vi "VALEW_Sensors_Hall.vi"(0 "GEA2 Reference In":refnum<k24>, 5 "GEA Inputs":T1={"Source"=228, "Destination"=35} {"Destination" format="%.0x"; "Source" format="%.0x"}, 7 "DAQmx Physical Channel":tag="9401_1/ctr2", 9 "Counter Terminal":tag="/9401_1/PFI4", 11 "Error In":errorcluster, 12 "Basket Test RPMs":dbl[](array[numeric])=[125.0, 500.0, 700.0], 13 "Max Error (RPM)":dbl=3.0, 14 "Standalone?":bool=TRUE) -> (4 "GEA2 Reference Out":refnum<k24>, 6 "Pass/Fail?":bool, 8 "Report Text":string, 15 "Error Out":errorcluster)   [LabVIEW 2016, in "2015 VA Washer.lvlib"]
doc: "This VI outputs the Test RPMs by generating a frequency that is 0.3 * Test RPM Value and verifies the Basket speed ERD is within the Max Error defined."
uses:
  Projects/2015 VA Washer.lvlib
  C:/Automation/DLLs/PC Dot Net/GeaCommunication.dll
  Common/LabVIEW GEA2 Toolkit/LabVIEW_GEA2_Toolkit.lvlibp/type defs/Source_Destination.ctl
  Common/LabVIEW GEA2 Toolkit/LabVIEW_GEA2_Toolkit.lvlibp/type defs/ERD Read Data In.ctl
  Common/LabVIEW GEA2 Toolkit/LabVIEW_GEA2_Toolkit.lvlibp/type defs/Data Type.ctl
  <vilib>/DAQmx/create/channels.llb/DAQmx Create Channel (CO-Pulse Generation-Frequency).vi
  <vilib>/DAQmx/configure/timing.llb/DAQmx Timing (Implicit).vi
  Common/LabVIEW GEA2 Toolkit/LabVIEW_GEA2_Toolkit.lvlibp
  <resource>/objmgr/daqmx.rc
panel:
  out "Lim_U_Basket Speed RPM":dbl[](array[numeric])
  out "Lim_L_Basket Speed RPM":dbl[](array[numeric])
  out "Basket Speed RPM":dbl[](array[numeric])
  out "Lim_L_Shaft Speed RPM":dbl[](array[numeric])
  out "Lim_U_Shaft Speed RPM":dbl[](array[numeric])
  out "Shaft Speed RPM":dbl[](array[numeric])
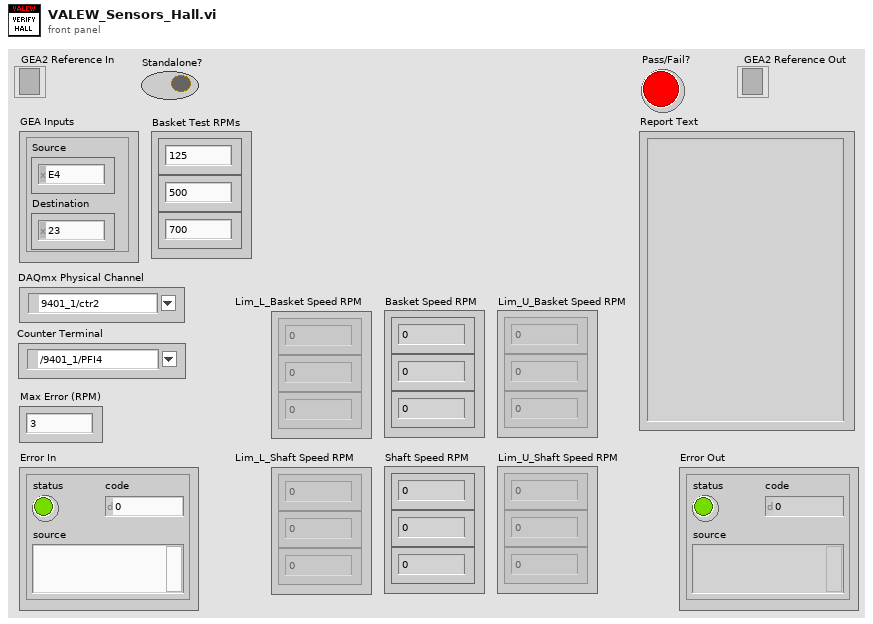
[diagram p1: front panel]
types:
  T1 = typedef "LabVIEW_GEA2_Toolkit.lvlibp/Source_Destination.ctl" = cluster{"Source":u8, "Destination":u8}
  T2 = typedef "LabVIEW_GEA2_Toolkit.lvlibp/ERD Read Data In.ctl" = cluster{"ERD Number":u16, "Data Type":T3}
  T3 = typedef "LabVIEW_GEA2_Toolkit.lvlibp/Data Type.ctl" = enum16{"string", "boolean", "uint8_t", "uint16_t", "uint32_t", "uint64_t", "int8_t", "int16_t", "int32_t", "int64_t"}
  T4 = typedef "LabVIEW_GEA2_Toolkit.lvlibp/ERD Read Data Out.ctl" = cluster{"ERD Number":u16, "Data":string}
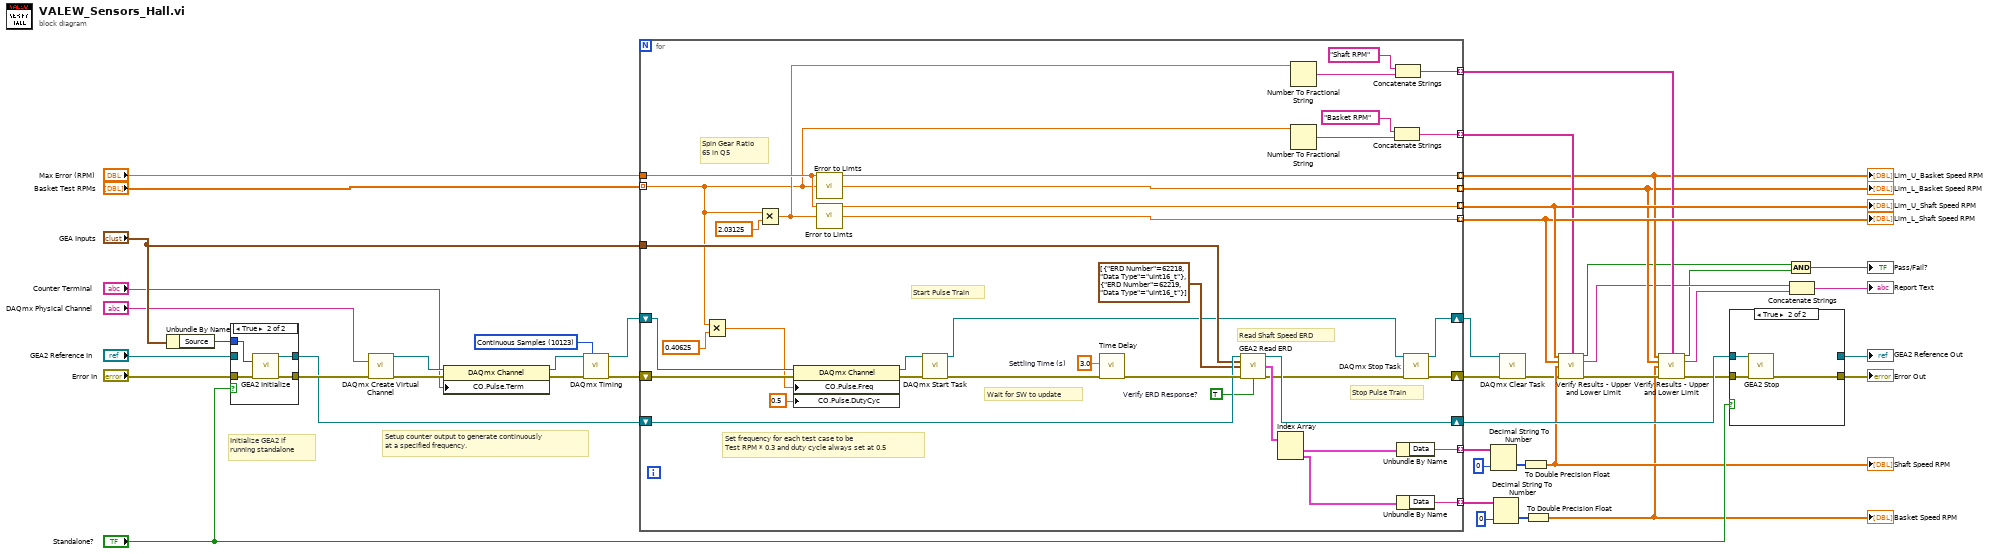
[diagram p0: block diagram]
diagram:
  w26 = 10123 items=["Finite Samples"=10178, "Continuous Samples"=10123, "Hardware Timed Single Point"=12522] ("sample mode")
  # "Setup counter output to generate continuously\nat a specified frequency."
  # "Initialize GEA2 if\nrunning standalone"
  n1 = Unbundle By Name("GEA Inputs") -> ("Source"=w38:u8)
  n2 = case shown="True" "Standalone?" {
    tunnel: "Error In" -> [w48 w52]
    tunnel: [w48 w51] -> w44
    tunnel: "GEA2 Reference In" -> [w47 _]
    tunnel: [w47 w50] -> w40
    tunnel: w38 -> [_ w49]
    frame False {
    }
    frame True {
      n3 = call "GEA2 Initialize.vi"("Source Address"=w49, "error in"=w52) -> ("GEA2 Reference Out"=w50:refnum<k24>, "error out"=w51:errorcluster)  [unwired: 11 in, 1 out]
    }
  }
  n4 = call-poly <vilib>:"DAQmx Create Virtual Channel.vi"("counter"="DAQmx Physical Channel", "error in"=w44) -> ("task out"=w31:refnum<k21>, "error out"=w32:errorcluster)  [unwired: 12 in]
  n5 = property class="DAQmx Channel"(reference=w31, error in=w32, "CO.Pulse.Term"="Counter Terminal") -> (reference out=w27:refnum<k21>, error out=w24:errorcluster)
  n6 = call-poly <vilib>:"DAQmx Timing.vi"("task/channels in"=w27, "sample mode"=w26, "error in"=w24) -> ("task out"=w25:refnum<k21>, "error out"=w23:errorcluster)  [unwired: 11 in]
  n7 = for {
    shift-right: [w79] -> w39
    shift-left: w40 -> [w88]
    shift-right: [w72] -> w43
    shift-left: w25 -> [w82]
    shift-right: [w73] -> w2
    shift-left: w23 -> [w81]
    tunnel: "GEA Inputs" -> [w87]
    tunnel: [w84] -> w36 mode=indexing
    tunnel: "Basket Test RPMs" -> [w53] mode=indexing
    tunnel: "Max Error (RPM)" -> [w60]
    tunnel: [w71] -> w20 mode=indexing
    tunnel: [w70] -> w21 mode=indexing
    tunnel: [w67] -> w18 mode=indexing
    tunnel: [w62] -> w12 mode=indexing
    tunnel: [w61] -> w11 mode=indexing
    tunnel: [w58] -> w15 mode=indexing
    tunnel: [w55] -> w13 mode=indexing
    w83 = TRUE  # Verify ERD Response?
    w90 = 3.0  # Settling Time (s)
    # "Spin Gear Ratio\n65 in Q5"
    # "Stop Pulse Train"
    # "Read Shaft Speed ERD"
    # "Wait for SW to update"
    # "Start Pulse Train"
    # "Set frequency for each test case to be\nTest RPM * 0.3 and duty cycle always set at 0.5"
    n8 = Multiply(x=w53, y=0.40625) -> (x*y=w63:dbl)
    n9 = Multiply(x=w53, y=2.03125) -> (x*y=w54:dbl)
    n10 = property class="DAQmx Channel"(reference=w82, error in=w81, "CO.Pulse.Freq"=w63, "CO.Pulse.DutyCyc"=0.5) -> (reference out=w75:refnum<k21>, error out=w76:errorcluster)
    n11 = call "Error to Limts.vi"("Error"=w60, "Value"=w53) -> ("Upper Limit"=w62:dbl, "Lower Limit"=w61:dbl)  [unwired: 12 in]
    n12 = call "Error to Limts.vi"("Error"=w60, "Value"=w54) -> ("Upper Limit"=w70:dbl, "Lower Limit"=w71:dbl)  [unwired: 12 in]
    n13 = call <vilib>:"DAQmx Start Task.vi"("task/channels in"=w75, "error in"=w76) -> ("task out"=w65:refnum<k21>, "error out"=w80:errorcluster)  [unwired: 12 in]
    n14 = call "Time Delay"("error in (no error)"=w80, "Delay Time (s)"=w90) -> ("error out"=w89:errorcluster)  [unwired: 9 in]
    n15 = call "GEA2 Read ERD.vi"("GEA2 Reference In"=w88, "GEA Inputs"=w87, "Read ERD List"=T2[] [{"ERD Number"=62218, "Data Type"=enum."uint16_t"}, {"ERD Number"=62219, "Data Type"=enum."uint16_t"}], "Error In"=w89, "Verify ERD Response?"=w83) -> ("GEA2 Reference Out"=w79:refnum<k24>, "ERD Data Out"=w86:T4[], "Error Out"=w74:errorcluster)  [unwired: 7 in, 1 out]
    n16 = Index Array(array=w86) -> (element #1=w85:T4, element #2=w59:T4)  [unwired: 2 in]
    n17 = Number To Fractional String(number=w54) -> (F-format string=w57:string)  [unwired: 3 in]
    n18 = Number To Fractional String(number=w53) -> (F-format string=w68:string)  [unwired: 3 in]
    n19 = Concatenate Strings("Basket RPM", w68) -> (w67:string)
    n20 = Concatenate Strings("Shaft RPM", w57) -> (w55:string)
    n21 = Unbundle By Name(w85) -> ("Data"=w84:string)
    n22 = Unbundle By Name(w59) -> ("Data"=w58:string)
    n23 = call <vilib>:"DAQmx Stop Task.vi"("task/channels in"=w65, "error in"=w74) -> ("task out"=w72:refnum<k21>, "error out"=w73:errorcluster)  [unwired: 12 in]
  }
  "Lim_U_Shaft Speed RPM" <- w21
  "Lim_L_Shaft Speed RPM" <- w20
  "Lim_U_Basket Speed RPM" <- w12
  "Lim_L_Basket Speed RPM" <- w11
  n24 = Decimal String To Number(string=w36, default (0L)=u16 0 ("default (0 I32)")) -> (number=w34:u16[])  [unwired: 1 in, 1 out]
  n25 = Decimal String To Number(string=w15, default (0L)=u16 0 ("default (0 I32)")) -> (number=w17:u16[])  [unwired: 1 in, 1 out]
  n26 = call <vilib>:"DAQmx Clear Task.vi"("task in"=w43, "error in"=w2) -> ("error out"=w3:errorcluster)  [unwired: 13 in]
  n27 = To Double Precision Float(number=w34) -> (double precision float=w19:dbl[])
  "Shaft Speed RPM" <- w19
  n28 = To Double Precision Float(number=w17) -> (double precision float=w10:dbl[])
  "Basket Speed RPM" <- w10
  n29 = call "Verify Results - Upper and Lower Limit.vi"("Upper Limits"=w21, "Array of Names"=w18, "Lower Limits"=w20, "Results"=w19, "Error In"=w3) -> ("Pass/Fail?"=w6:bool, "Report Text"=w8:string, "Error Out"=w14:errorcluster)  [unwired: 7 in, 1 out]
  n30 = call "Verify Results - Upper and Lower Limit.vi"("Upper Limits"=w12, "Array of Names"=w13, "Lower Limits"=w11, "Results"=w10, "Error In"=w14) -> ("Pass/Fail?"=w5:bool, "Report Text"=w7:string, "Error Out"=w1:errorcluster)  [unwired: 7 in, 1 out]
  n31 = case shown="True" "Standalone?" {
    tunnel: [w91 w95] -> w41
    tunnel: w39 -> [w92 w93]
    tunnel: [w92 _] -> w42
    tunnel: w1 -> [w91 w94]
    frame False {
    }
    frame True {
      n32 = call "GEA2 Stop.vi"("GEA2 Reference In"=w93, "Error In"=w94) -> ("Error Out"=w95:errorcluster)  [unwired: 13 in]
    }
  }
  "Error Out" <- w41
  "GEA2 Reference Out" <- w42
  n33 = And(x=w6, y=w5) -> (x .and. y?=→"Pass/Fail?":bool)
  n34 = Concatenate Strings(w8, w7) -> (→"Report Text":string)
